vi "Get Active Channels.vi"(8 "error in":errorcluster, 11 "custom device ref":T1=18446744073709551615 format="%.0x") -> (0 "error out":errorcluster, 2 "active channels":T4(array[cluster]), 3 "custom device ref out":T1 format="%.0x")   [LabVIEW 2020, in "AIM ARINC 429 Scripting.lvlib"]
doc: "Returns configuration for all active ports within the <b>custom device ref</b>."
uses:
  AIM ARINC 429 Scripting.lvlib
  <vilib>/NI VeriStand/Custom Device API/Custom Device Item Ref.ctl
  Shared/Direction.ctl
  Shared/Transfer Speed.ctl
  <vilib>/NI VeriStand/Custom Device API/Custom Device API.lvlib
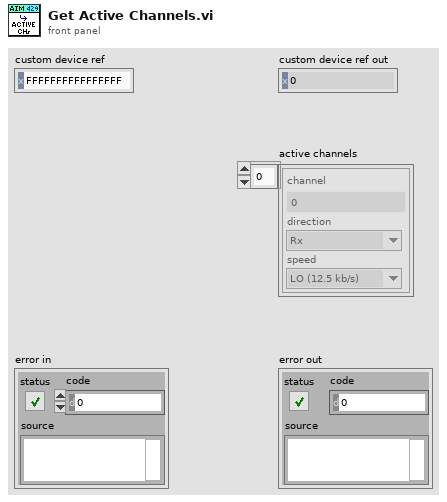
[diagram p1: front panel]
types:
  T1 = typedef "Custom Device API.lvlib/Custom Device Item Ref.ctl" = u64
  T2 = typedef "Direction.ctl" = enum16{"Rx", "Tx"}
  T3 = typedef "Transfer Speed.ctl" = enum16{"LO (12.5 kb/s)", "HI (100 kb/s)"}
  T4 = cluster{"channel":u8, "direction":T2, "speed":T3}[]
  T5 = cluster{"channel":u8, "direction":T2, "speed":T3}
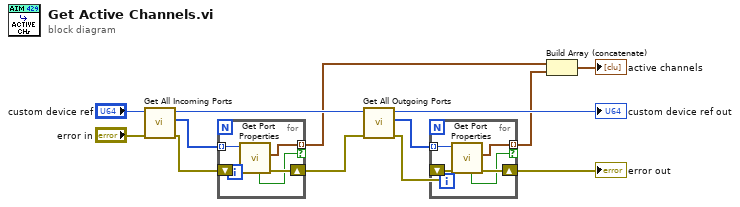
[diagram p0: block diagram]
diagram:
  n1 = call "Get All Incoming Ports.vi"("error in"="error in", "custom device ref"="custom device ref") -> ("error out"=w11:errorcluster, "incoming ports"=w12:T1[], "custom device ref out"=w13:T1)  [unwired: 7 in]
  n2 = for {
    tunnel: w12 -> [w18] mode=indexing
    shift-right: [w16] -> w7
    shift-left: w11 -> [w17]
    tunnel: [w15] -> w2 mode=indexing if=w14
    n3 = call "Get Port Properties.vi"("error in"=w17, "port ref in"=w18) -> ("error out"=w16:errorcluster, "channel configuration"=w15:T5, "found?"=w14:bool)  [unwired: 6 in, 1 out]
  }
  n4 = call "Get All Outgoing Ports.vi"("error in"=w7, "custom device ref"=w13) -> ("error out"=w5:errorcluster, "outgoing ports"=w6:T1[], "custom device ref out"=→"custom device ref out":T1)  [unwired: 7 in]
  n5 = for {
    tunnel: w6 -> [w23] mode=indexing
    shift-right: [w21] -> w4
    shift-left: w5 -> [w22]
    tunnel: [w20] -> w1 mode=indexing if=w19
    n6 = call "Get Port Properties.vi"("error in"=w22, "port ref in"=w23) -> ("error out"=w21:errorcluster, "channel configuration"=w20:T5, "found?"=w19:bool)  [unwired: 6 in, 1 out]
  }
  "error out" <- w4
  n7 = Build Array (concatenate)(w2, w1) -> (→"active channels":T4)
